vi "Handle Error (User).vi"(8 "error in":errorcluster, 11 "Node in":refnum<class "BLS Cycler Template.lvclass">) -> (0 "error out":errorcluster, 3 "Node out":refnum<class "BLS Cycler Template.lvclass">)   [LabVIEW 2023, in "BLS Cycler Template.lvlib" / "BLS Cycler Template.lvclass"]
uses:
  BLS Cycler Template.lvclass
  BLS Cycler Template.lvclass/BLS Cycler Template.ctl
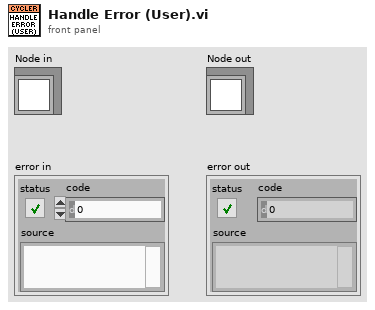
[diagram p1: front panel]
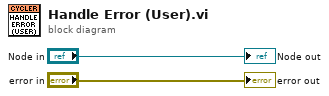
[diagram p0: block diagram]
diagram:
  "error out" <- "error in"
  "Node out" <- "Node in"
